vi "Get SubpanelVI Info.vi"(8 "error in (no error)":errorcluster, 11 "VacuumLine Configuration in":refnum<class "VacuumLine Configuration.lvclass">) -> (0 "error out":errorcluster, 1 "Array of Subpanel VI data":T1[](array[typedef]), 2 "Array of Category string":string[](array[string]), 3 "VacuumLine Configuration out":refnum<class "VacuumLine Configuration.lvclass">)   [LabVIEW 2016, in "Hardware.lvlib" / "VacuumLine.lvlib" / "VacuumLine Configuration.lvclass"]
uses:
  <userlib>/Common Components/Hardware/Abstract System/VacuumLine/VacuumLine Config/VacuumLine Configuration.lvclass
  <userlib>/Configuration Dialog Actor/Methods/Data Retrieved by Lookup Table.ctl
  <userlib>/Configuration Dialog Actor/Configuration.lvclass
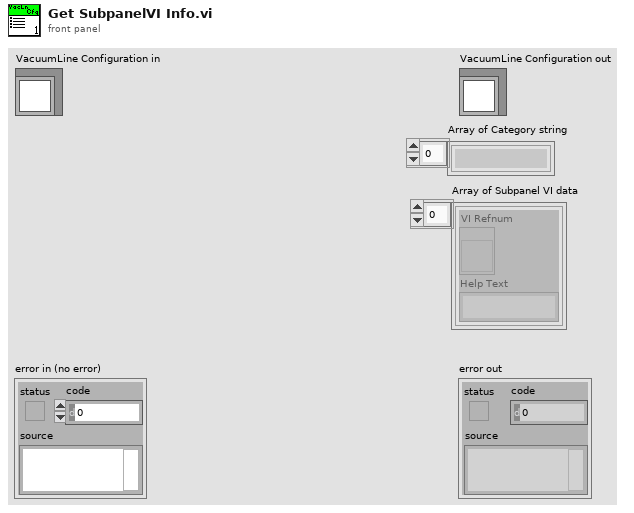
[diagram p1: front panel]
types:
  T1 = typedef "Configuration.lvlib/Configuration.lvclass/Data Retrieved by Lookup Table.ctl" = cluster{"VI Refnum":refnum<vi>, "Help Text":string}
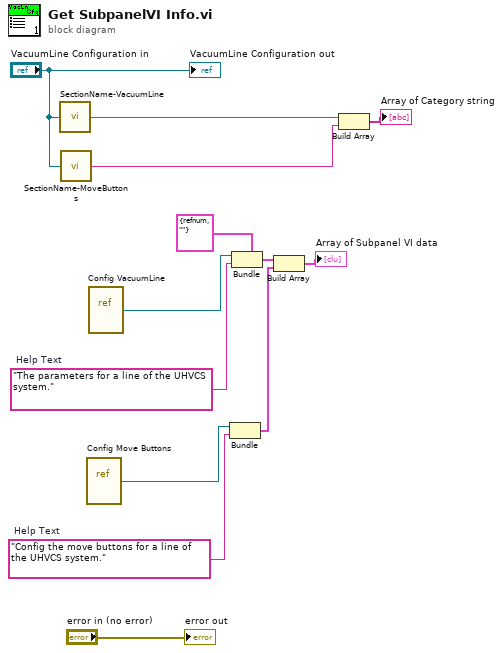
[diagram p0: block diagram]
diagram:
  w4 = "Config the move buttons for a line of the UHVCS system."  # Help Text
  w7 = "The parameters for a line of the UHVCS system."  # Help Text
  n1 = call <userlib>:"SectionName-VacuumLine.vi"("VacuumLine Configuration in"="VacuumLine Configuration in") -> ("SectionName"=w6:string)
  n2 = call <userlib>:"SectionName-MoveButtons.vi"("VacuumLine Configuration in"="VacuumLine Configuration in") -> ("SectionName"=w2:string)
  n3 = vi-ref <userlib>:"Config Move Buttons.vi"() -> (w5:refnum<vi>)
  n4 = vi-ref <userlib>:"Config VacuumLine.vi"() -> (w8:refnum<vi>)
  n5 = Bundle(w5, "Help Text"=w4) -> (w3:cluster{refnum<vi>, "Help Text":string})  [unwired: 1 in]
  n6 = Bundle(cluster=T1 {"VI Refnum"=refnum, "Help Text"=""} ("output cluster"), "VI Refnum"=w8, "Help Text"=w7) -> (w9:T1)
  n7 = Build Array(w9, w3) -> (→"Array of Subpanel VI data":T1[])
  n8 = Build Array(w6, w2) -> (→"Array of Category string":string[])
  "error out" <- "error in (no error)"
  "VacuumLine Configuration out" <- "VacuumLine Configuration in"
